vi "Read Encoders.vi"(9 "Reset Encoders":bool, 11 "Encoder":string="My Counter RefNum") -> (1 "Debug":i32, 2 "Counts":i32, 3 "Orig Count":i32)   [LabVIEW 2014]
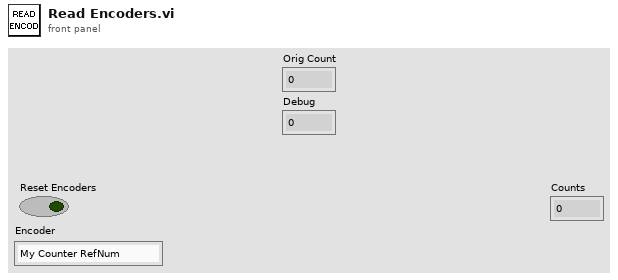
[diagram p1: front panel]
types:
  T1 = typedef "WPI_CounterDevRef.ctl" = cluster{"DevStatus":errorcluster, "CntIndex":T2}
  T2 = typedef "FPGA_CounterCtrSystemIndex.ctl" = enum8{"Ctr 0", "Ctr 1", "Ctr 2", "Ctr 3", "Ctr 4", "Ctr 5", "Ctr 6", "Ctr 7", "Invalid"}
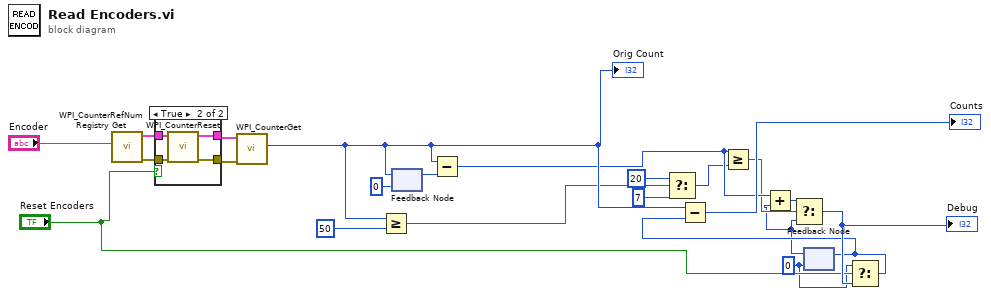
[diagram p0: block diagram]
diagram:
  w7 = 0
  n1 = call <vilib>:"WPI_CounterRefNum Registry Get.vi"("refnum name"="Encoder") -> ("error out"=w20:errorcluster, "CounterDevRef"=w19:T1)  [unwired: 9 in]
  n2 = case shown="True" "Reset Encoders" {
    tunnel: [w24 w28] -> w22
    tunnel: [w23 w27] -> w21
    tunnel: w19 -> [w24 w26]
    tunnel: w20 -> [w23 w25]
    frame False {
    }
    frame True {
      n3 = call <vilib>:"WPI_CounterReset.vi"("error in (no error)"=w25, "CounterDevRef in"=w26) -> ("error out"=w27:errorcluster, "CounterDevRef out"=w28:T1)  [unwired: 8 in]
    }
  }
  n4 = call <vilib>:"WPI_CounterGet.vi"("error in (no error)"=w21, "CounterDevRef in"=w22) -> ("Value"=w16:i32)  [unwired: 4 in, 5 out]
  "Orig Count" <- w16
  n5 = Greater Or Equal?(x=w16, y=50) -> (x >= y?=w9:bool)
  n6 = feedback #1(0 ("Value")) -> (w11:i32)
  n7 = feedback-in #1(w16) -> ()
  n8 = Subtract(x=w16, y=w11) -> (x-y=w10:i32)
  n9 = Select(t=20 ("f"), s=w9, f=7 ("y")) -> (s? t:f=w3:i32)
  n10 = Greater Or Equal?(x=w10, y=w3) -> (x >= y?=w8:bool)
  n11 = feedback #2(w7) -> (w4:i32)
  n12 = Add(x=w10, y=w4) -> (x+y=w5:i32)
  n13 = Select(t=w5, s=w8, f=w4) -> (s? t:f=w15:i32)
  "Debug" <- w15
  n14 = Select(t=w7, s="Reset Encoders", f=w15) -> (s? t:f=w6:i32)
  n15 = Subtract(x=w16, y=w6) -> (x-y=→"Counts":i32)
  n16 = feedback-in #2(w6) -> ()
